vi "programa 1.vi"() -> ()   [LabVIEW 2011]
uses:
  Control del programa1.ctl
panel:
  out "Array":T1(array[cluster]) {"Temp3" scale=0.0..60.0; "Temp2" scale=0.0..60.0; "Temp1" scale=0.0..60.0}
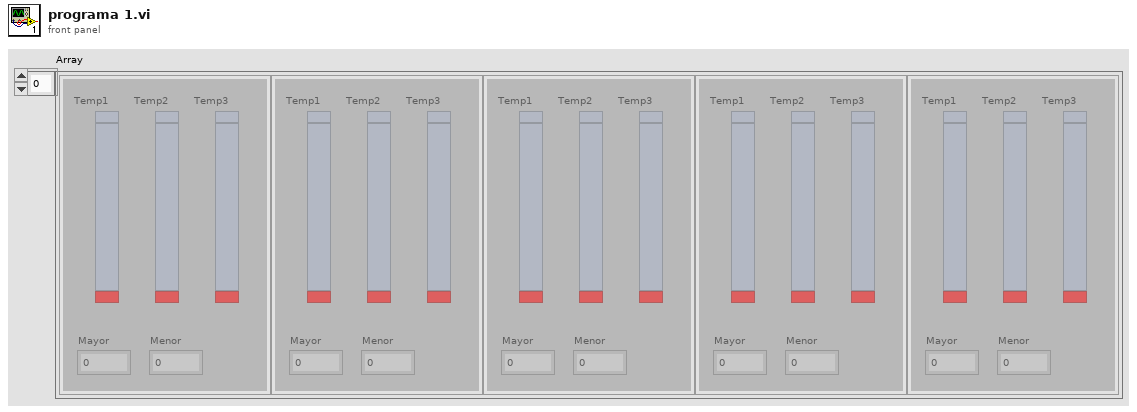
[diagram p1: front panel]
types:
  T1 = cluster{"Temp1":i32, "Temp2":i32, "Temp3":i32, "Mayor":dbl, "Menor":dbl}[]
  T2 = typedef "Control del programa1.ctl" = enum16{"Iniciar Arreglos", "Ingresar Temps", "Obtener Max y Min", "Finalizar"}
  T3 = cluster{"Temp1":i32, "Temp2":i32, "Temp3":i32, "Mayor":dbl, "Menor":dbl}
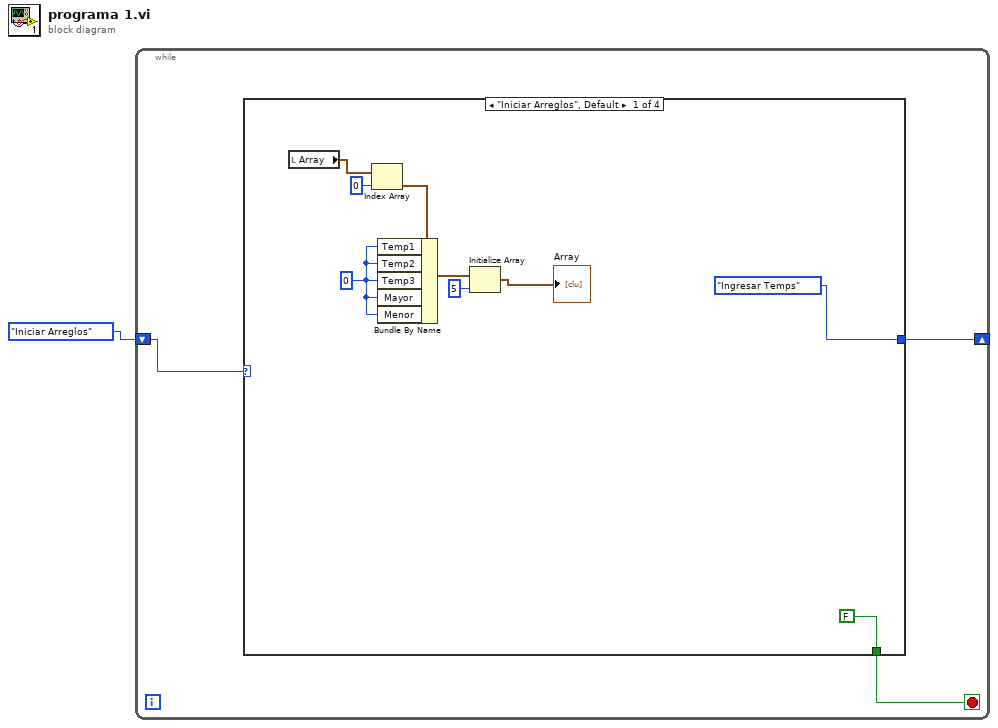
[diagram p0: block diagram]
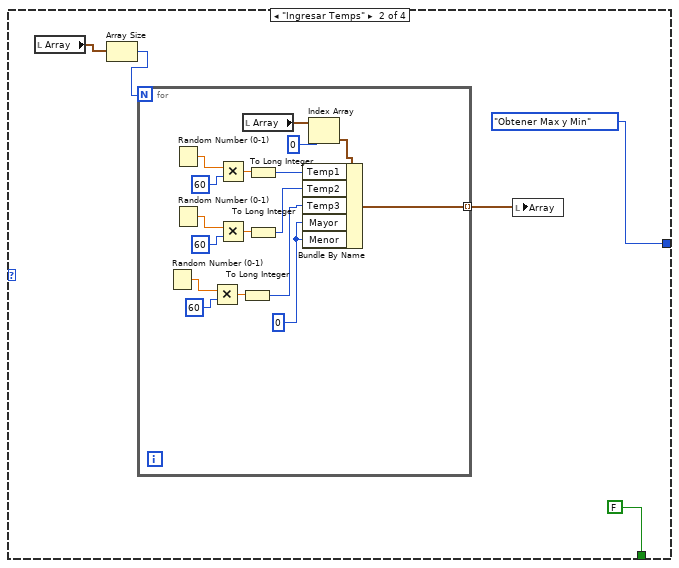
[diagram p2: hidden frame]
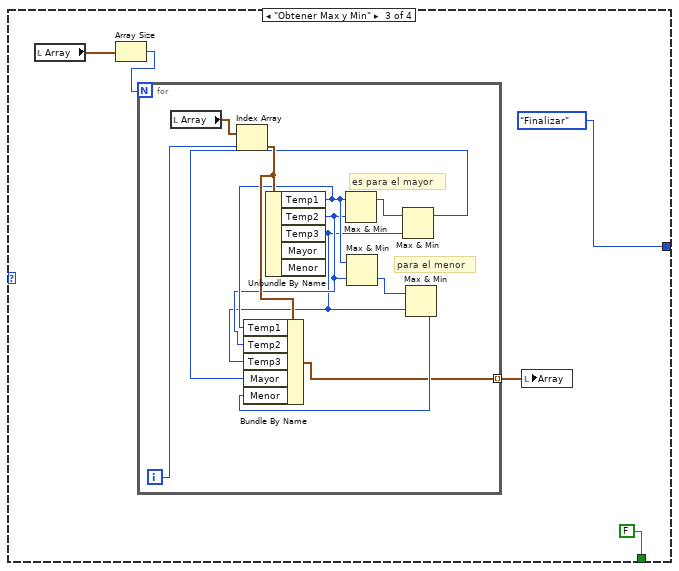
[diagram p3: hidden frame]
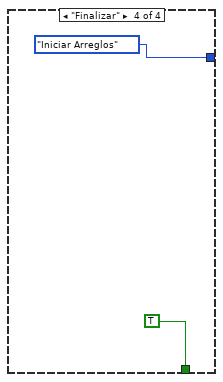
[diagram p4: hidden frame]
diagram:
  n1 = while {
    shift-right: [w3] -> _
    shift-left: Control_del_programa1."Iniciar Arreglos" -> [w4]
    stop <- w2 stop-if-true
    n2 = case shown="\"Iniciar Arreglos\", Default" w4 {
      tunnel: [Control_del_programa1."Ingresar Temps" Control_del_programa1."Obtener Max y Min" Control_del_programa1."Finalizar" Control_del_programa1."Iniciar Arreglos"] -> w3
      tunnel: [FALSE FALSE FALSE TRUE] -> w2
      frame "Iniciar Arreglos", Default {
        w8 = 0
        n3 = local read "Array"() -> (w11:T1)
        n4 = Index Array "Index Array"(array=w11, index=0) -> (element=w9:T3)
        n5 = Bundle By Name "Bundle By Name"(cluster=w9, "Temp1"=w8, "Temp2"=w8, "Temp3"=w8, "Mayor"=w8, "Menor"=w8) -> (w12:T3)
        n6 = Initialize Array "Initialize Array"(w12, 5 ("dimension size")) -> (→"Array":T1)
      }
      frame "Ingresar Temps" {
        n7 = local read "Array"() -> (w18:T1)
        n8 = Array Size(array=w18) -> (size(s)=w17:i32)
        n9 = for {
          N: w17 -> [_]
          tunnel: [w19] -> w16 mode=indexing
          w20 = 0
          n10 = Random Number (0-1)() -> (number: 0 to 1=w23:dbl)
          n11 = Random Number (0-1)() -> (number: 0 to 1=w29:dbl)
          n12 = Random Number (0-1)() -> (number: 0 to 1=w28:dbl)
          n13 = Multiply(x=w23, y=60) -> (x*y=w25:dbl)
          n14 = Multiply(x=w29, y=60) -> (x*y=w32:dbl)
          n15 = Multiply(x=w28, y=60) -> (x*y=w26:dbl)
          n16 = To Long Integer(number=w25) -> (32bit integer=w21:i32)
          n17 = local read "Array"() -> (w35:T1)
          n18 = To Long Integer(number=w32) -> (32bit integer=w31:i32)
          n19 = To Long Integer(number=w26) -> (32bit integer=w22:i32)
          n20 = Index Array "Index Array"(array=w35, index=0) -> (element=w33:T3)
          n21 = Bundle By Name(cluster=w33, "Temp1"=w31, "Temp2"=w22, "Temp3"=w21, "Mayor"=w20, "Menor"=w20) -> (w19:T3)
        }
        n22 = local write "Array"(w16) -> ()
      }
      frame "Obtener Max y Min" {
        n23 = local read "Array"() -> (w40:T1)
        n24 = Array Size(array=w40) -> (size(s)=w39:i32)
        n25 = for {
          N: w39 -> [_]
          tunnel: [w41] -> w38 mode=indexing
          i -> [w50]
          # "para el menor"
          # "es para el mayor"
          n26 = local read "Array"() -> (w51:T1)
          n27 = Index Array "Index Array"(array=w51, index=w50) -> (element=w47:T3)
          n28 = Unbundle By Name(w47) -> ("Temp1"=w44:i32, "Temp2"=w43:i32, "Temp3"=w42:i32)  [unwired: 2 out]
          n29 = Max & Min(x=w44, y=w43) -> (max(x,y)=w49:i32)  [unwired: 1 out]
          n30 = Max & Min(x=w44, y=w43) -> (min(x,y)=w48:i32)  [unwired: 1 out]
          n31 = Max & Min(x=w49, y=w42) -> (max(x,y)=w45:i32)  [unwired: 1 out]
          n32 = Max & Min(x=w48, y=w42) -> (min(x,y)=w46:i32)  [unwired: 1 out]
          n33 = Bundle By Name(cluster=w47, "Temp1"=w44, "Temp2"=w43, "Temp3"=w42, "Mayor"=w45, "Menor"=w46) -> (w41:T3)
        }
        n34 = local write "Array"(w38) -> ()
      }
      frame "Finalizar" {
      }
    }
  }
